vi "TW_HTTPErr_old.vi"(8 "error in (no error)":errorcluster, 10 "HTTP Code":i32, 11 "Comm":T1) -> ()   [LabVIEW 2019]
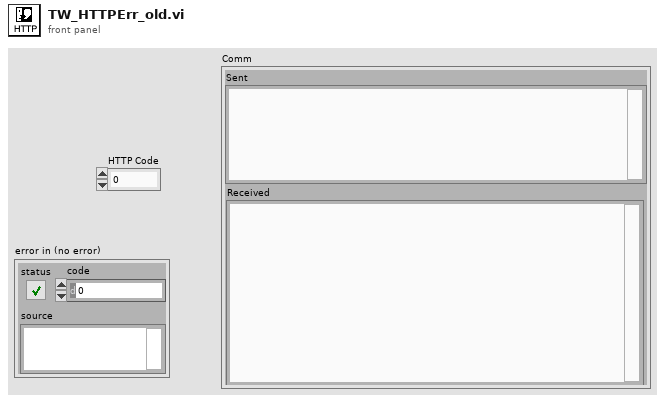
[diagram p1: front panel]
types:
  T1 = cluster{"url":string, "sent headers":string, "sent body":string, "headers":string, "body":string, "Sent":string, "Received":string}
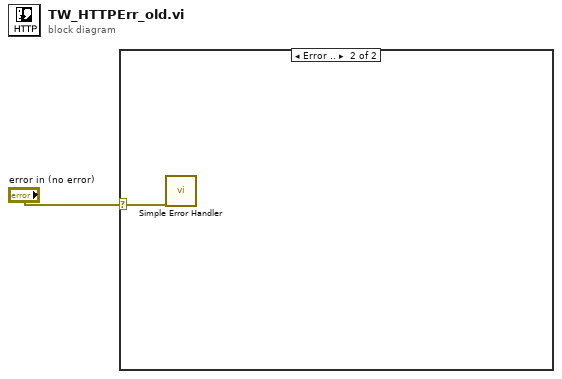
[diagram p0: block diagram]
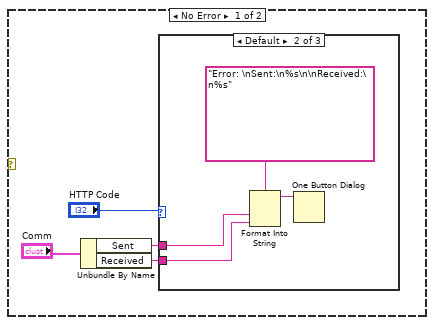
[diagram p2: hidden frame]
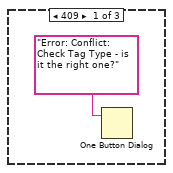
[diagram p3: hidden frame]
diagram:
  n1 = case shown="Error .." "error in (no error)" {
    selector: "error in (no error)" -> [_ w11]
    frame No Error {
      n2 = Unbundle By Name("Comm") -> ("Sent"=w3:string, "Received"=w2:string)
      n3 = case shown="Default" "HTTP Code" {
        tunnel: w3 -> [_ w8 _]
        tunnel: w2 -> [_ w7 _]
        frame 409 {
          n4 = One Button Dialog(message="Error: Conflict: Check Tag Type - is it the right one?") -> ()  [unwired: 1 in, 1 out]
        }
        frame Default {
          n5 = Format Into String(format string="Error: \nSent:\n%s\n\nReceived:\n%s" ("message"), w8, w7) -> (resulting string=w9:string)  [unwired: 2 in, 1 out]
          n6 = One Button Dialog(message=w9) -> ()  [unwired: 1 in, 1 out]
        }
        frame 200 {
        }
      }
    }
    frame Error {
      n7 = call <vilib>:"Simple Error Handler.vi"("error in (no error)"=w11) -> ()  [unwired: 4 in, 5 out]
    }
  }
